vi "testTriggerGenUserEventServerAandB.vi"(8 "error in":errorcluster) -> (0 "error out":errorcluster)   [LabVIEW 2018]
doc: "Test the generic user event sent from servers A and B."
uses:
  src/TcpServerBase/typedef/connStatusCluster.ctl
  <vilib>/addons/_JKI Toolkits/Caraya/classes/Assert/Assert Equal Value_Variant.vi
  src/TcpServerCmd/TcpServerCmd.lvclass
  <vilib>/addons/_JKI Toolkits/Caraya/classes/Assert/Assert.lvclass
  src/TcpServerBase/TcpServerBase.lvclass
  <vilib>/addons/_JKI Toolkits/Caraya/classes/Test/Test.lvclass
panel:
  out "connStatusB":bool[](array[boolean])
  out "connStatusA":bool[](array[boolean])
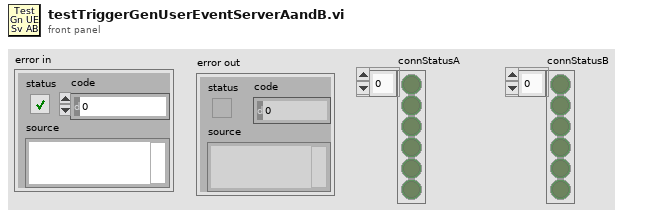
[diagram p1: front panel]
types:
  T1 = typedef "TcpServerBase.lvclass/connStatusCluster.ctl" = cluster{"connStatus":bool, "message":string}
  T2 = cluster{"CmdRead":refnum<user-event>, "EvtRead":refnum<user-event>, "GenRead":refnum<user-event>}
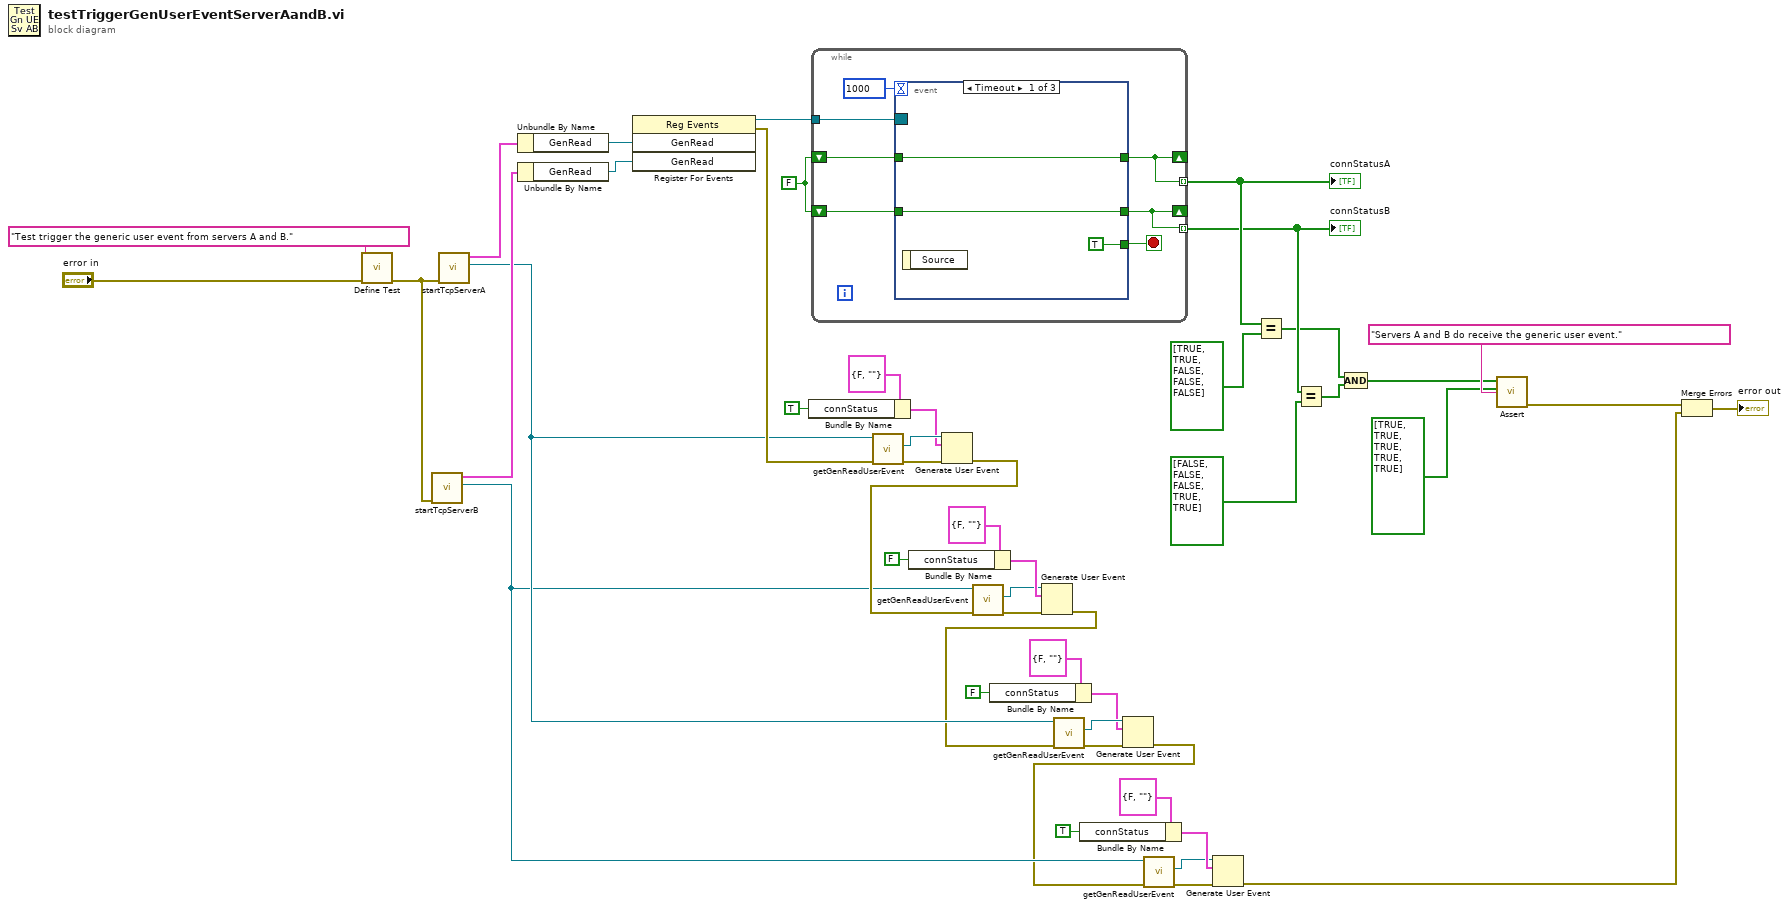
[diagram p0: block diagram]
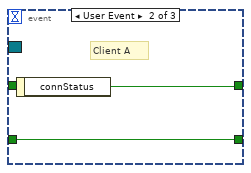
[diagram p2: hidden frame]
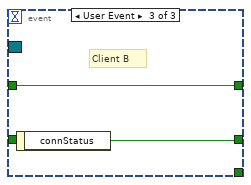
[diagram p3: hidden frame]
diagram:
  w47 = FALSE ("connStatus")
  n1 = call <vilib>:"Define Test.vi"("error in (no error)"="error in", "Label (VI Title)"="Test trigger the generic user event from servers A and B.") -> ("error out"=w27:errorcluster)  [unwired: 9 in]
  n2 = call "startTcpServerB.vi"("error in (no error)"=w27) -> ("TcpServer out"=w13:refnum<class "TcpServer.lvclass">, "UserEvents"=w26:T2)  [unwired: 8 in, 1 out]
  n3 = call "startTcpServerA.vi"("error in (no error)"=w27) -> ("TcpServer out"=w14:refnum<class "TcpServer.lvclass">, "UserEvents"=w46:T2)  [unwired: 8 in, 1 out]
  n4 = Unbundle By Name(w46) -> ("GenRead"=w39:refnum<user-event>)
  n5 = Unbundle By Name(w26) -> ("GenRead"=w25:refnum<user-event>)
  n6 = register-events(w39, w25) -> (reference out=w38:refnum<event-registration>, error out=w34:errorcluster)  [unwired: 2 in]
  n7 = Bundle By Name(cluster=T1 {"connStatus"=FALSE, "message"=""} ("event data"), "connStatus"=TRUE) -> (w35:T1)
  n8 = while {
    shift-right: [w49] -> _
    shift-left: w47 -> [w53]
    shift-right: [w48] -> _
    shift-left: w47 -> [w52]
    tunnel: w38 -> [w50]
    tunnel: [w49] -> w6 mode=indexing
    tunnel: [w48] -> w4 mode=indexing
    stop <- w51 stop-if-true
    n9 = event shown="[0] Timeout" {
      selector: w50 -> [_ _ _]
      dyn-events: _ -> [_ _ _]
      timeout: 1000 -> [_ _ _]
      tunnel: [w57 w59 w60] -> w49
      tunnel: [w56 w58 w61] -> w48
      tunnel: w53 -> [w57 _ w60]
      tunnel: w52 -> [w56 w58 _]
      tunnel: [TRUE _ _] -> w51
      event Timeout {
        n10 = event-data() -> ()  [unwired: 1 in, 1 out]
      }
      event User Event {
        # "Client A"
        n11 = event-data() -> ("connStatus"=w59:bool)  [unwired: 1 in]
      }
      event User Event {
        # "Client B"
        n12 = event-data() -> ("connStatus"=w61:bool)  [unwired: 1 in]
      }
    }
  }
  "connStatusA" <- w6
  "connStatusB" <- w4
  n13 = call "getGenReadUserEvent.vi"("error in (no error)"=w34, "TcpServer in"=w14) -> ("error out"=w44:errorcluster, "GenRead"=w45:refnum<user-event>)  [unwired: 7 in, 1 out]
  n14 = Bundle By Name(cluster=T1 {"connStatus"=FALSE, "message"=""} ("event data"), "connStatus"=FALSE) -> (w32:T1)
  n15 = Generate User Event(user event=w45, event data cluster=w35, error in=w44) -> (error out=w33:errorcluster)  [unwired: 1 in, 1 out]
  n16 = call "getGenReadUserEvent.vi"("error in (no error)"=w33, "TcpServer in"=w13) -> ("error out"=w29:errorcluster, "GenRead"=w28:refnum<user-event>)  [unwired: 7 in, 1 out]
  n17 = Bundle By Name(cluster=T1 {"connStatus"=FALSE, "message"=""} ("event data"), "connStatus"=FALSE) -> (w20:T1)
  n18 = Generate User Event(user event=w28, event data cluster=w32, error in=w29) -> (error out=w12:errorcluster)  [unwired: 1 in, 1 out]
  n19 = call "getGenReadUserEvent.vi"("error in (no error)"=w12, "TcpServer in"=w14) -> ("error out"=w23:errorcluster, "GenRead"=w24:refnum<user-event>)  [unwired: 7 in, 1 out]
  n20 = Bundle By Name(cluster=T1 {"connStatus"=FALSE, "message"=""} ("event data"), "connStatus"=TRUE) -> (w19:T1)
  n21 = Generate User Event(user event=w24, event data cluster=w20, error in=w23) -> (error out=w11:errorcluster)  [unwired: 1 in, 1 out]
  n22 = call "getGenReadUserEvent.vi"("error in (no error)"=w11, "TcpServer in"=w13) -> ("error out"=w16:errorcluster, "GenRead"=w15:refnum<user-event>)  [unwired: 7 in, 1 out]
  n23 = Generate User Event(user event=w15, event data cluster=w19, error in=w16) -> (error out=w10:errorcluster)  [unwired: 1 in, 1 out]
  n24 = Equal?(x=w6, y=bool[] [TRUE, TRUE, FALSE, FALSE, FALSE] ("Array 4")) -> (x = y?=w2:bool[])
  n25 = Equal?(x=w4, y=bool[] [FALSE, FALSE, FALSE, TRUE, TRUE] ("Array 3")) -> (x = y?=w1:bool[])
  n26 = Compound Arithmetic op=AND(w2, w1) -> (w8:bool[])
  n27 = call-poly <vilib>:"Assert.vi"("Label"="Servers A and B do receive the generic user event.", "Y"=bool[] [TRUE, TRUE, TRUE, TRUE, TRUE] ("y"), "X"=w8) -> ("error out"=w43:errorcluster)  [unwired: 8 in]
  n28 = Merge Errors(w43, w10) -> (→"error out":errorcluster)
